vi "Fix data type.vi"(8 "error in (no error)":errorcluster, 10 "Binary?":bool, 11 "Workspace":path) -> (0 "error out":errorcluster)   [LabVIEW 2019]
panel:
  out "Files corected":i32
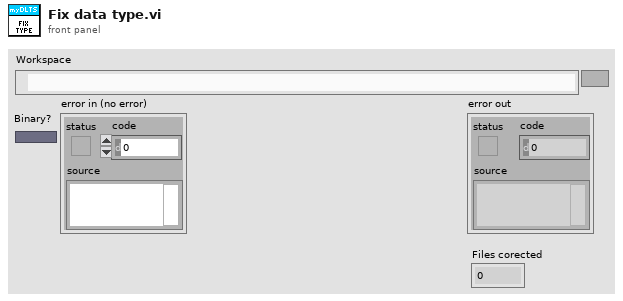
[diagram p1: front panel]
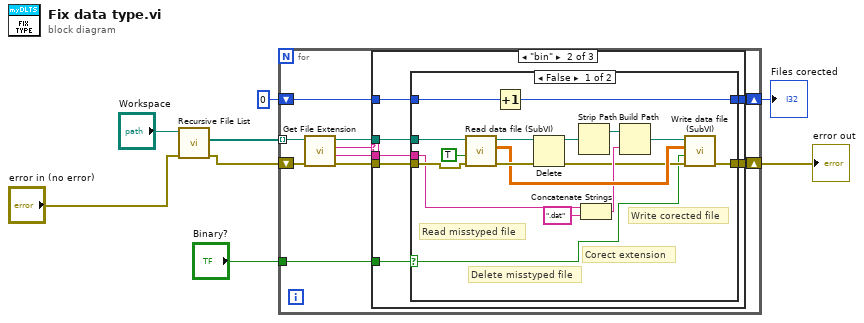
[diagram p0: block diagram]
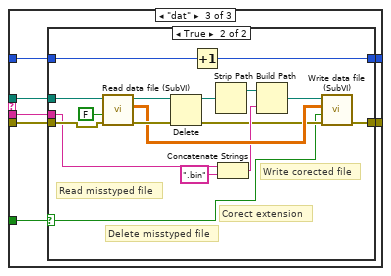
[diagram p4: hidden frame]
diagram:
  n1 = call <vilib>:"Recursive File List.vi"("error in (no error)"="error in (no error)", "Folder Path"="Workspace") -> ("error out"=w5:errorcluster, "All Files in Dir"=w7:path[])  [unwired: 5 in, 3 out]
  n2 = for {
    tunnel: w7 -> [w18] mode=indexing
    tunnel: "Binary?" -> [w13]
    shift-right: [w12] -> w3
    shift-left: w5 -> [w16]
    shift-right: [w9] -> w1
    shift-left: 0 -> [w10]
    n3 = call <vilib>:"Get File Extension.vi"("error in (no error)"=w16, "file"=w18) -> ("error out"=w14:errorcluster, "filename without extension"=w17:string, "lowercase file extension"=w11:string, "dup file"=w15:path)  [unwired: 5 in, 1 out]
    n4 = case shown="\"bin\"" w11 {
      tunnel: w17 -> [_ w25 w51]
      tunnel: w15 -> [_ w26 w52]
      tunnel: w14 -> [w20 w24 w50]
      tunnel: w13 -> [_ w27 w53]
      tunnel: [w20 w23 w49] -> w12
      tunnel: w10 -> [w19 w22 w48]
      tunnel: [w19 w21 w47] -> w9
      frame "", Default {
      }
      frame "bin" {
        n5 = case shown="False" w27 {
          selector: w27 -> [w30 _]
          tunnel: w26 -> [w44 _]
          tunnel: w25 -> [w36 _]
          tunnel: w24 -> [w42 w46]
          tunnel: [w32 w46] -> w23
          tunnel: w22 -> [w29 w45]
          tunnel: [w28 w45] -> w21
          frame False {
            # "Write corected file"
            # "Corect extension"
            # "Delete misstyped file"
            # "Read misstyped file"
            n6 = call "Read data file (SubVI).vi"("error in"=w42, "Binary"=TRUE, "file path in"=w44) -> ("error out"=w41:errorcluster, "2D data"=w39:dbl[][], "file path out"=w40:path)  [unwired: 6 in]
            n7 = Increment(x=w29) -> (x+1=w28:i32)
            n8 = Delete(path (use dialog)=w40, error in=w41) -> (deleted path=w38:path, error out=w31:errorcluster)  [unwired: 3 in, 1 out]
            n9 = Strip Path(path=w38) -> (stripped path=w37:path)  [unwired: 1 out]
            n10 = Concatenate Strings(w36, ".dat" ("string")) -> (w35:string)
            n11 = Build Path(base path=w37, name or relative path=w35) -> (appended path=w34:path)
            n12 = call "Write data file (SubVI).vi"("error in"=w31, "Binary"=w30, "2D data"=w39, "file path in"=w34) -> ("error out"=w32:errorcluster)  [unwired: 6 in, 1 out]
          }
          frame True {
          }
        }
      }
      frame "dat" {
        n13 = case shown="True" w53 {
          selector: w53 -> [_ w58]
          tunnel: w52 -> [_ w72]
          tunnel: w51 -> [_ w64]
          tunnel: w50 -> [w55 w70]
          tunnel: [w55 w60] -> w49
          tunnel: w48 -> [w54 w57]
          tunnel: [w54 w56] -> w47
          frame False {
          }
          frame True {
            # "Write corected file"
            # "Corect extension"
            # "Delete misstyped file"
            # "Read misstyped file"
            n14 = call "Read data file (SubVI).vi"("error in"=w70, "Binary"=FALSE, "file path in"=w72) -> ("error out"=w69:errorcluster, "2D data"=w67:dbl[][], "file path out"=w68:path)  [unwired: 6 in]
            n15 = Delete(path (use dialog)=w68, error in=w69) -> (deleted path=w66:path, error out=w59:errorcluster)  [unwired: 3 in, 1 out]
            n16 = Increment(x=w57) -> (x+1=w56:i32)
            n17 = Strip Path(path=w66) -> (stripped path=w65:path)  [unwired: 1 out]
            n18 = Concatenate Strings(w64, ".bin" ("string")) -> (w63:string)
            n19 = Build Path(base path=w65, name or relative path=w63) -> (appended path=w62:path)
            n20 = call "Write data file (SubVI).vi"("error in"=w59, "Binary"=w58, "2D data"=w67, "file path in"=w62) -> ("error out"=w60:errorcluster)  [unwired: 6 in, 1 out]
          }
        }
      }
    }
  }
  "error out" <- w3
  "Files corected" <- w1
